vi "스마트 공장_프로젝트_3조.vi"() -> ()   [LabVIEW 2021]
uses:
  <vilib>/Utility/sysdir.llb/System Directory Type.ctl
  <vilib>/DAQmx/read.llb/DAQmx Read (Counter DBL 1Chan 1Samp).vi
  <vilib>/DAQmx/read.llb/DAQmx Read (Analog 1D Wfm NChan NSamp).vi
  <vilib>/Analysis/baseanly.llb/Mean (DBL).vi
  <vilib>/DAQmx/write.llb/DAQmx Write (Counter Frequency 1Chan 1Samp).vi
  <vilib>/DAQmx/create/channels.llb/DAQmx Create Channel (AI-Voltage-Basic).vi
  <vilib>/DAQmx/configure/timing.llb/DAQmx Timing (Sample Clock).vi
  <vilib>/DAQmx/create/channels.llb/DAQmx Create Channel (CI-Count Edges).vi
  <vilib>/DAQmx/create/channels.llb/DAQmx Create Channel (CO-Pulse Generation-Frequency).vi
  <vilib>/DAQmx/configure/timing.llb/DAQmx Timing (Implicit).vi
  <vilib>/DAQmx/miscellaneous.llb/DAQmx Fill In Error Info.vi
  <vilib>/measure/maspectr.llb/FFT Power Spectrum for N Chan.vi
  <resource>/objmgr/daqmx.rc
  <vilib>/measure/NI_MAPro.lvlib
  <vilib>/Analysis/NI_AALBase.lvlib
panel:
  in  "Axis_Factor":u16(ring) items=["X", "Y", "Z"]
  out "시간 문자열":string
  out "Temp":dbl format="%0.2f"
  out "Distance":dbl caption="DISTANCE" format="%0.2f"
  out "Z":dbl format="%0.2f"
  out "Y":dbl format="%0.2f"
  out "X":dbl format="%0.2f"
  out "t0":timestamp
  out "추가된 배열":waveform(dbl)[](array[waveform])
  out "크기":i32
  out "배열":waveform(dbl)[](array[waveform])
  out "MAX-DISTANCE":dbl
  out "웨이브폼 그래프":cluster{"f0":dbl, "df":dbl, "magnitude":dbl[]}[](graph)
  out "data":dbl caption="RPM" format="%0.2f"
  out "CONNECT":bool
  in  "stop":bool
  in  "start":bool
  in  "exit":bool
  in  "File Name":string
  in  "LIMITED-DISTANCE":dbl
  in  "디스플레이 영역(s)":dbl
  in  "Window":u16(ring)
  in  "Number of average":u16(ring)
  in  "Average mode":u16(ring)
  in  "회전당 펄스":dbl
  in  "TEMP-OFFSET":dbl
  in  "TEMP-FACTOR":dbl
  in  "DISTANCE-OFFSET":dbl
  in  "DISTANCE-FACTOR":dbl
  in  "AXIS-OFFSET":dbl
  out "웨이브폼 차트":waveform(dbl)[](graph)
  # "SMART-FACTORY"
  # "Time Domain Graph"
  # "Frequency Domain Graph"
  # "SETTING"
  # "DATA"
  # "Time Domain"
  # "Waveform graph"
  # "Time domain vertical bar"
  # "Frequency Domain"
  # "Window"
  # "Average Parameter"
  # "config data"
  # "calibration"
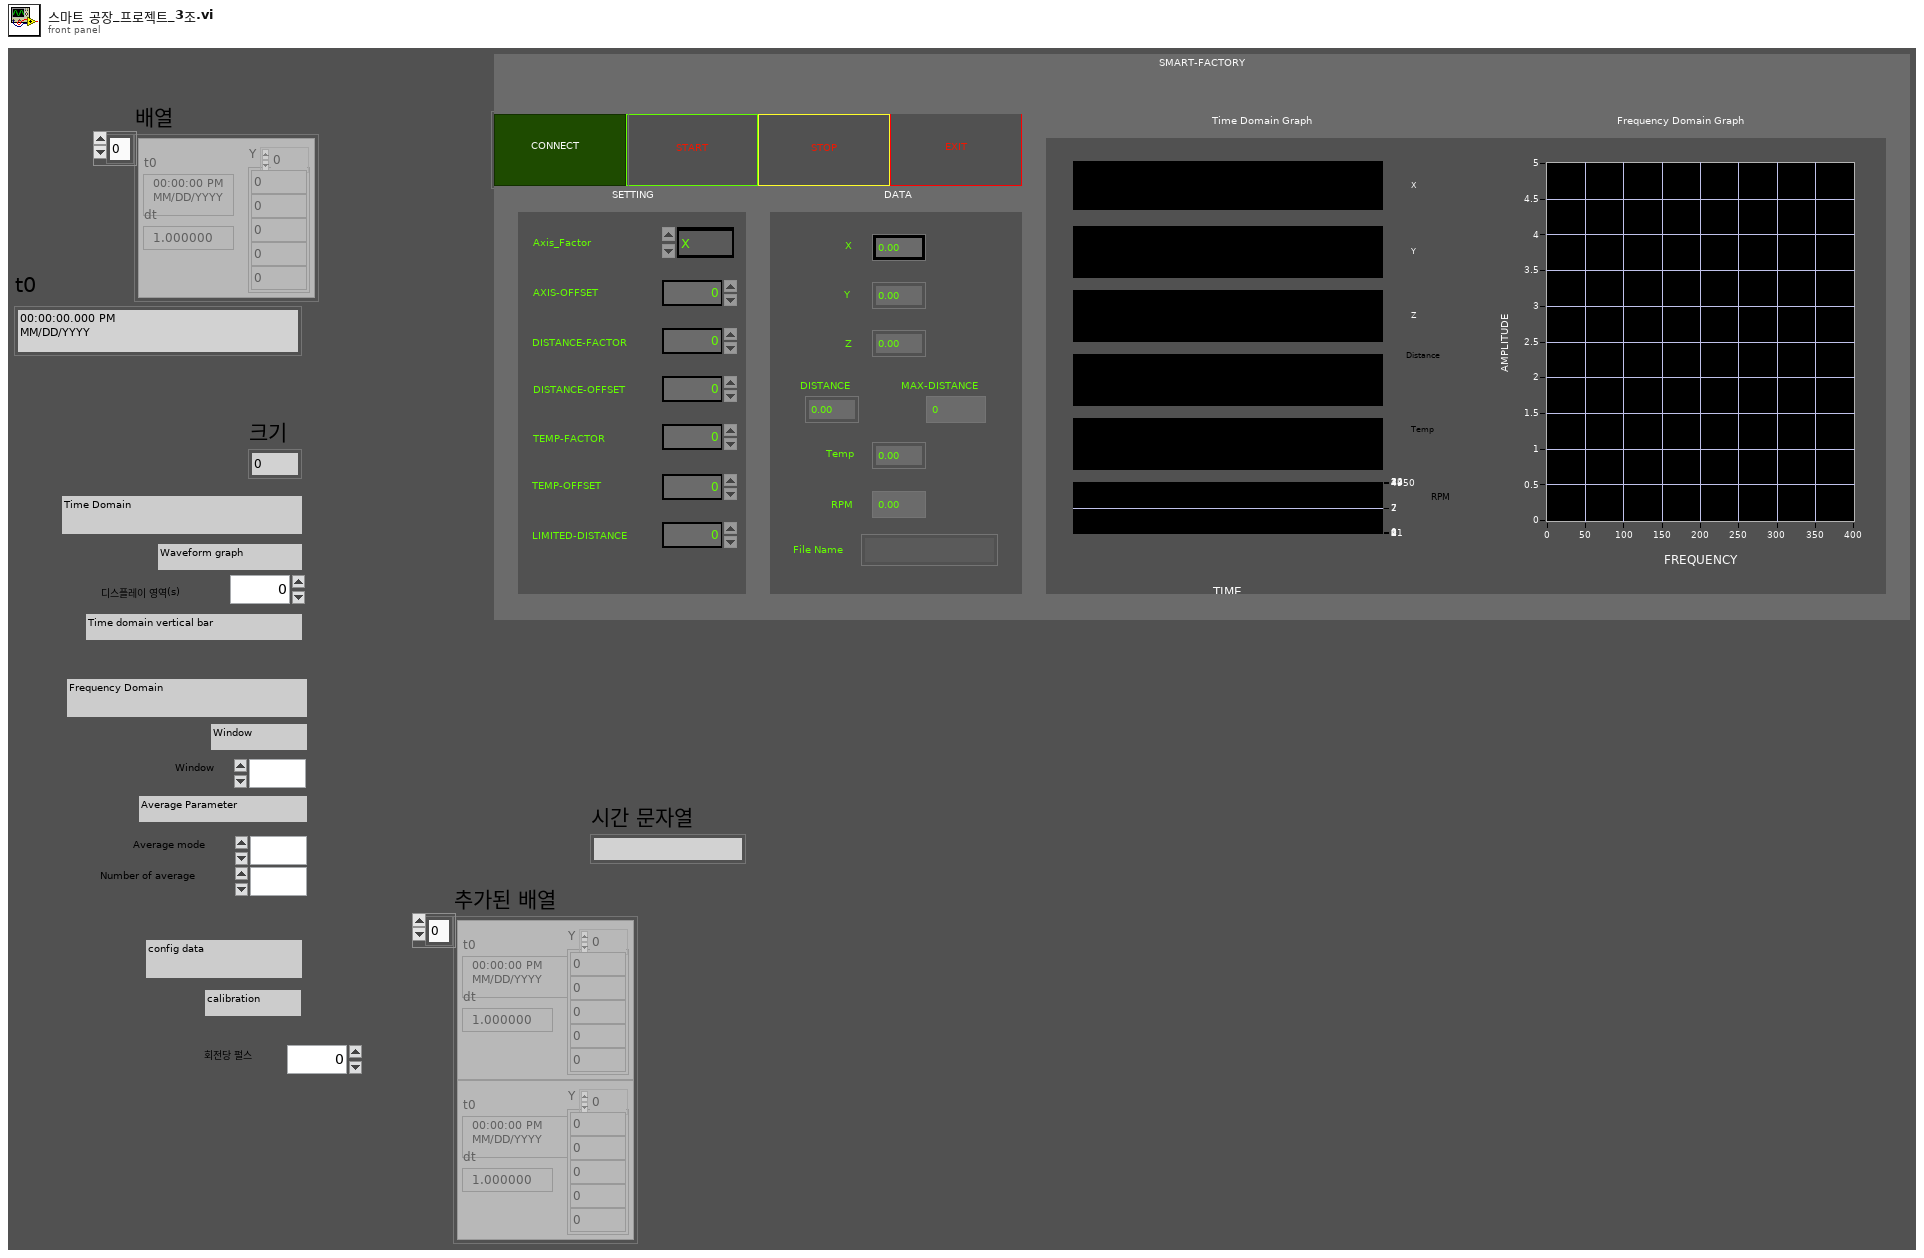
[diagram p1: front panel]
types:
  T1 = typedef "공장.ctl" = enum16{"초기화", "Ready", "Start", "Stop", "Exit"}
  T2 = cluster{"x_time(s)":i32, "y_time(s)":i32, "z_time(s)":i32, T1, "temp_time(s)":i32, "rpm_time(s)":i32, "x_data":i32, "y_data":i32, "z_data":i32, "distance_time(s)":i32, "temp_data":i32, "rpm_data":i32, "distance_data":i32, "MOTOR_PULSE":refnum<k21>, "AI_SIGNAL":refnum<k21>, "DI_SIGNAL":refnum<k21>, "CONNECT_LED":bool, "저장 파일":refnum<k34>, "system":bool, "카운트":dbl}
  T3 = enum16{"open", "open or create", "create or replace", "create", "open (read-only)"}
  T4 = enum8{"Enabled", "Disabled", "Disabled and Grayed Out"}
  T5 = typedef "System Directory Type.ctl" = i32
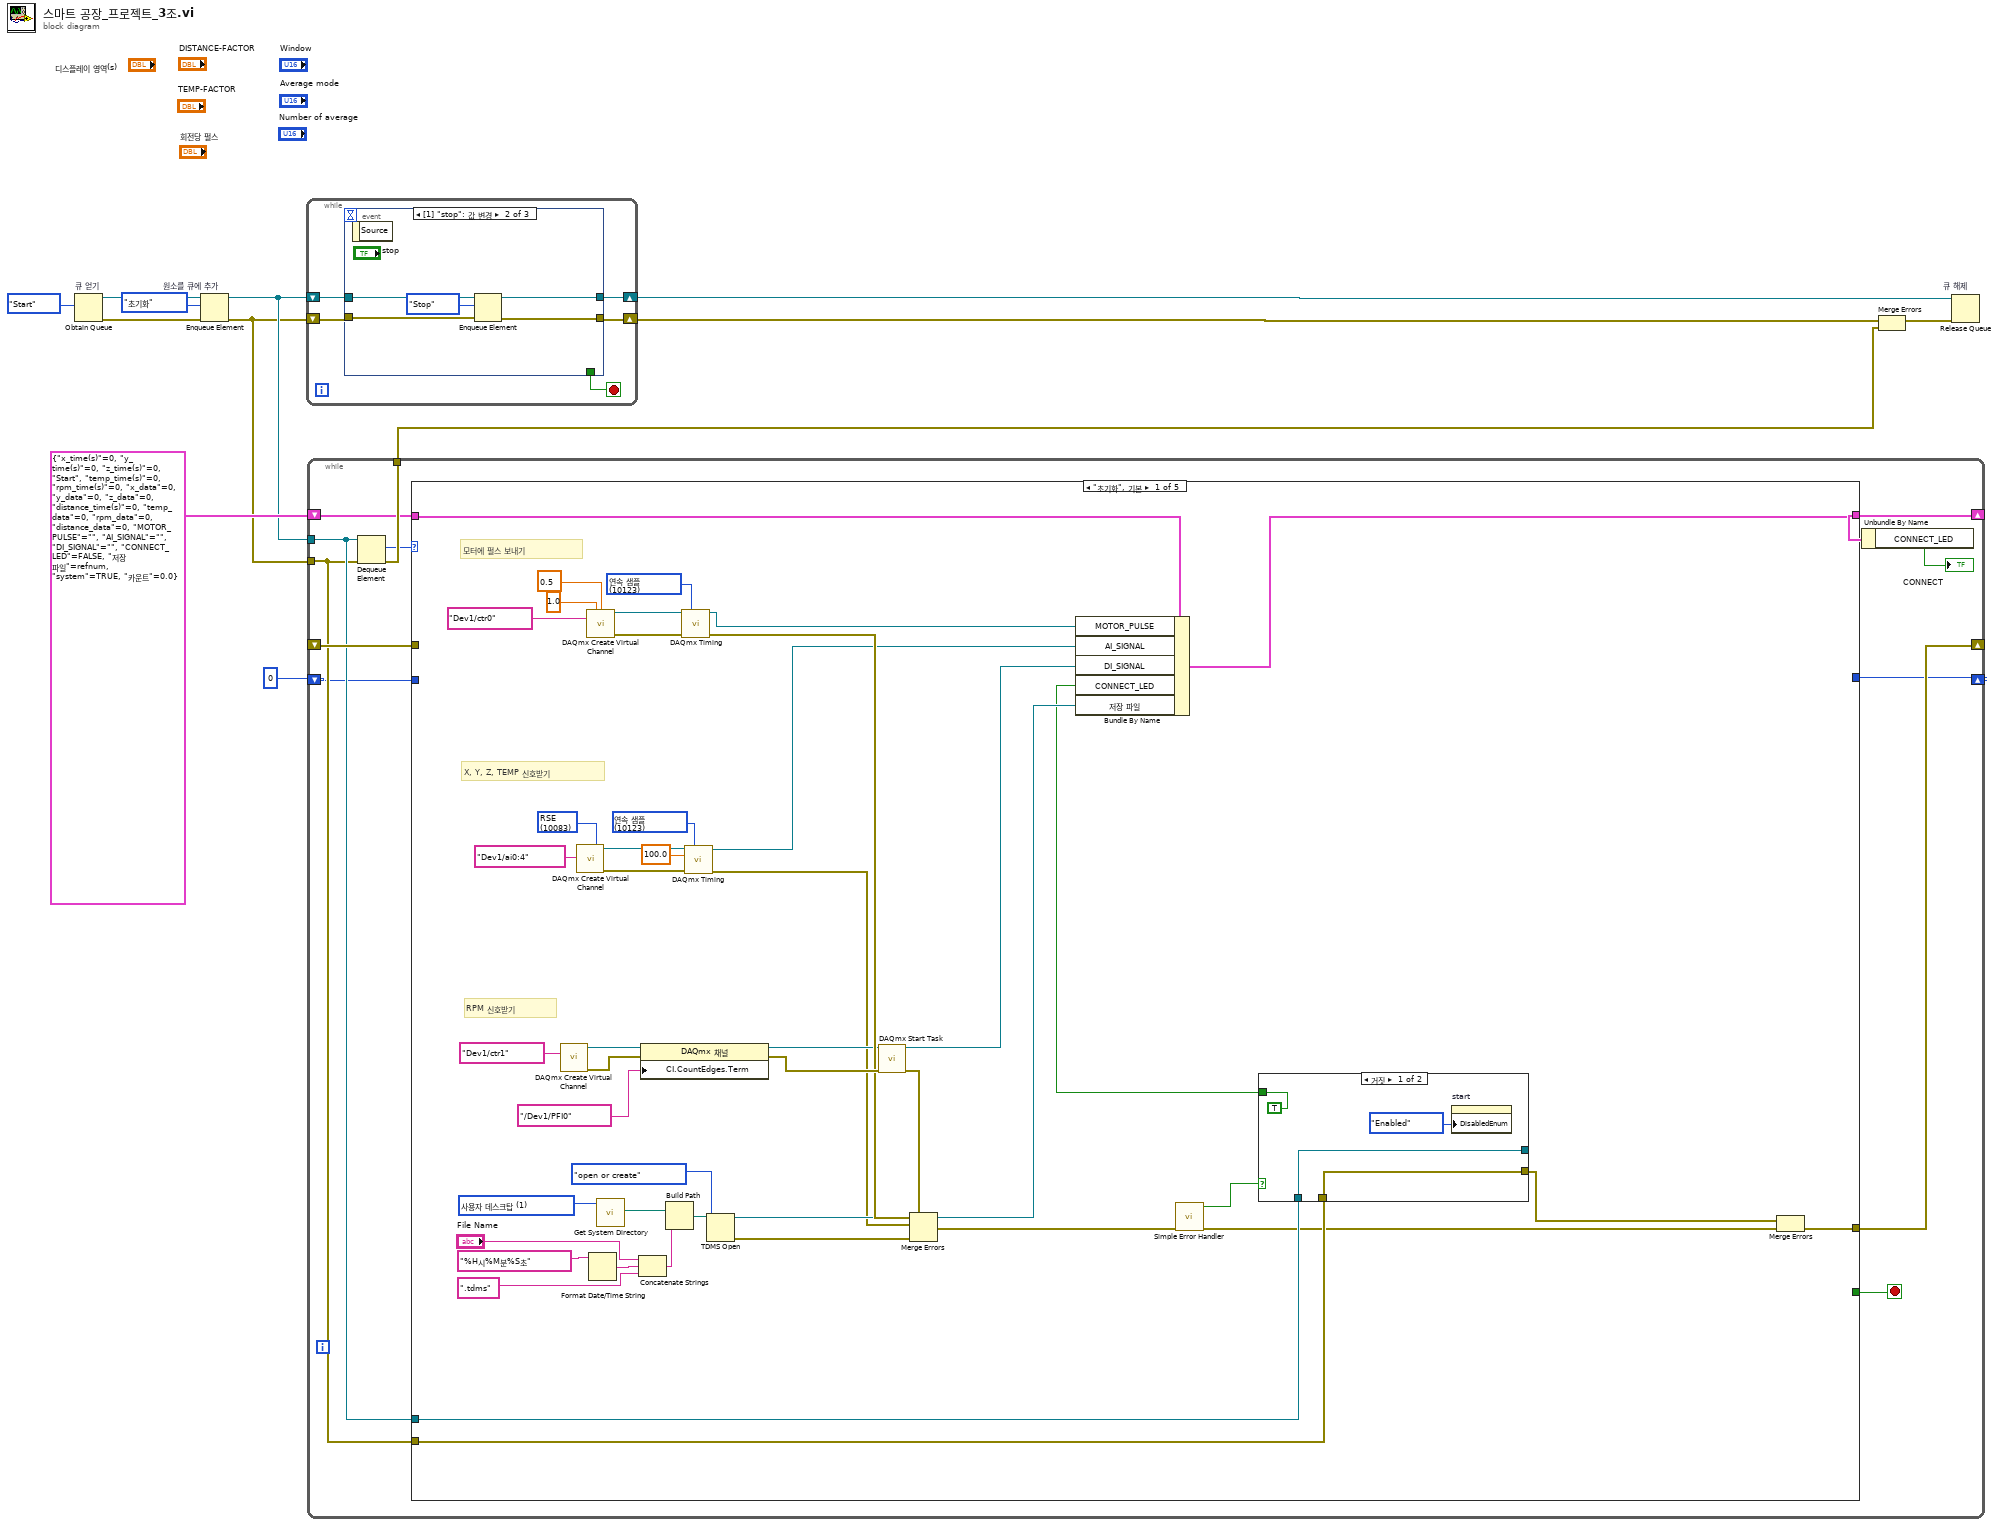
[diagram p0: block diagram]
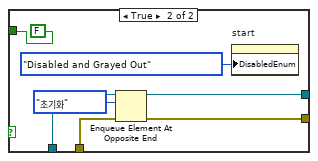
[diagram p2: hidden frame]
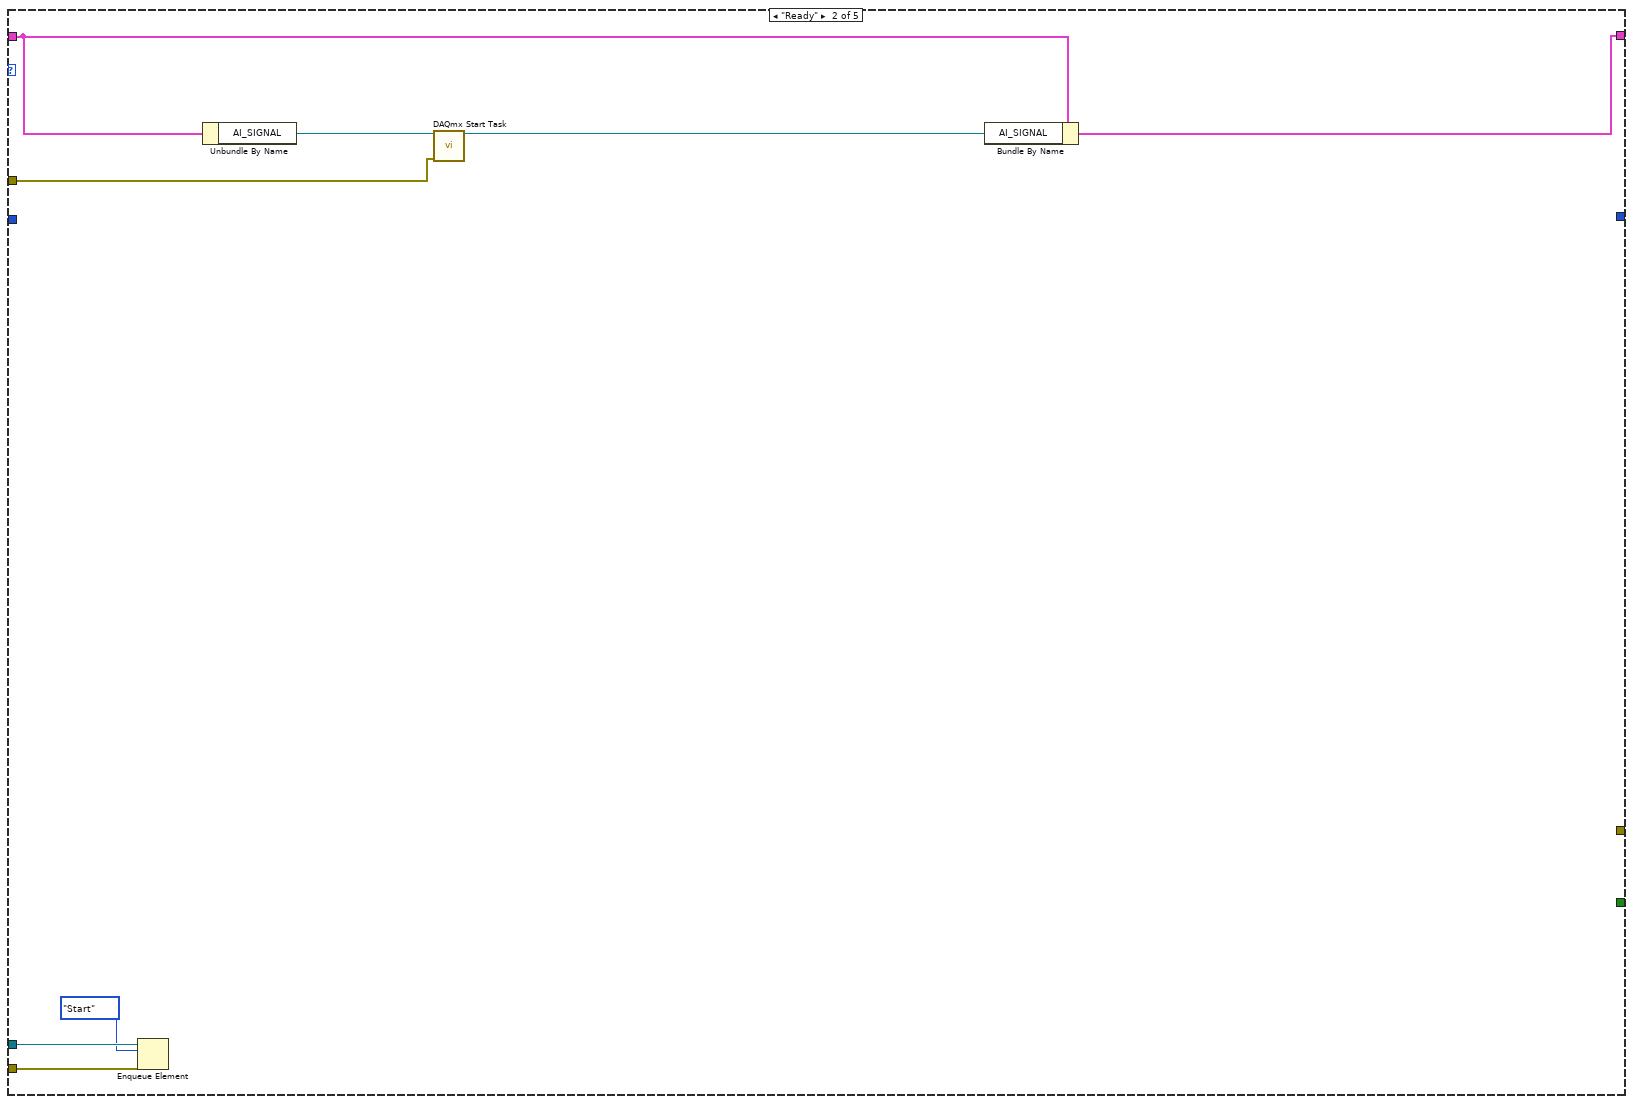
[diagram p3: hidden frame]
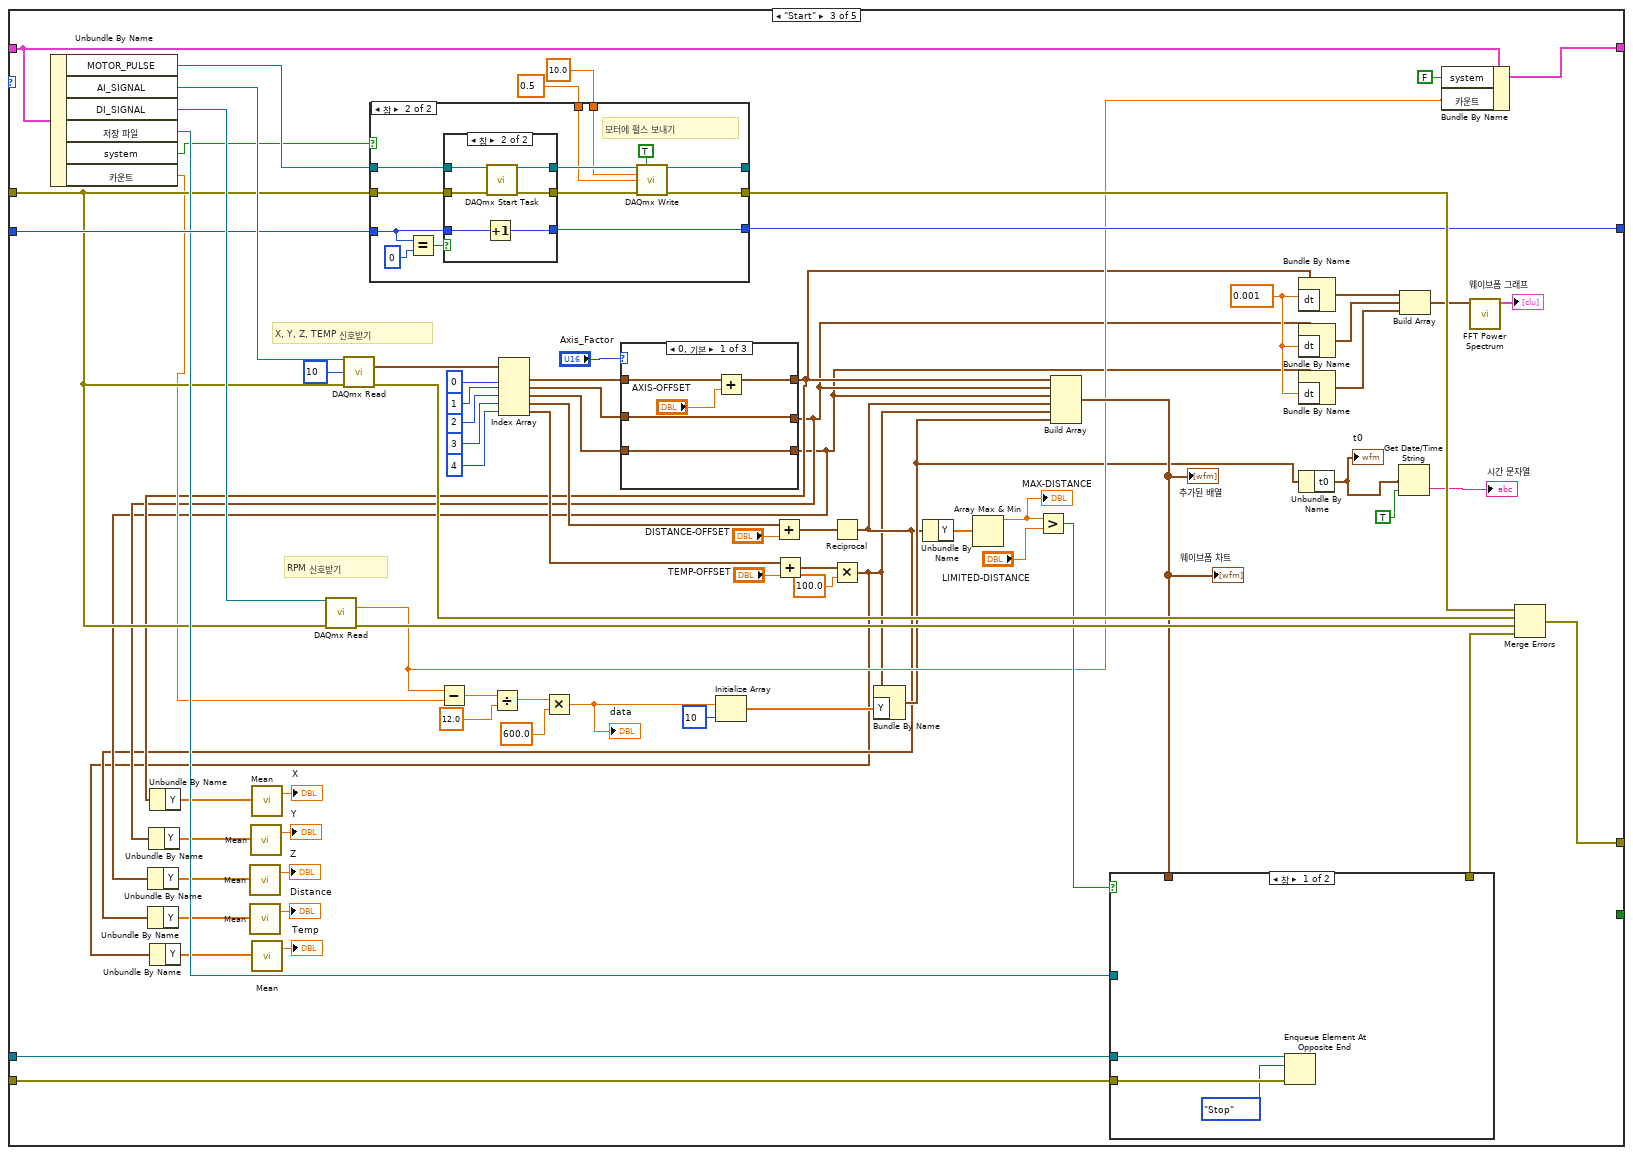
[diagram p4: hidden frame]
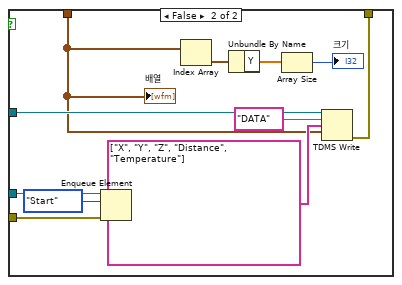
[diagram p7: hidden frame]
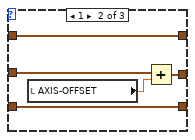
[diagram p8: hidden frame]
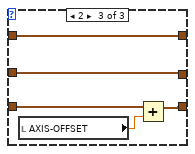
[diagram p9: hidden frame]
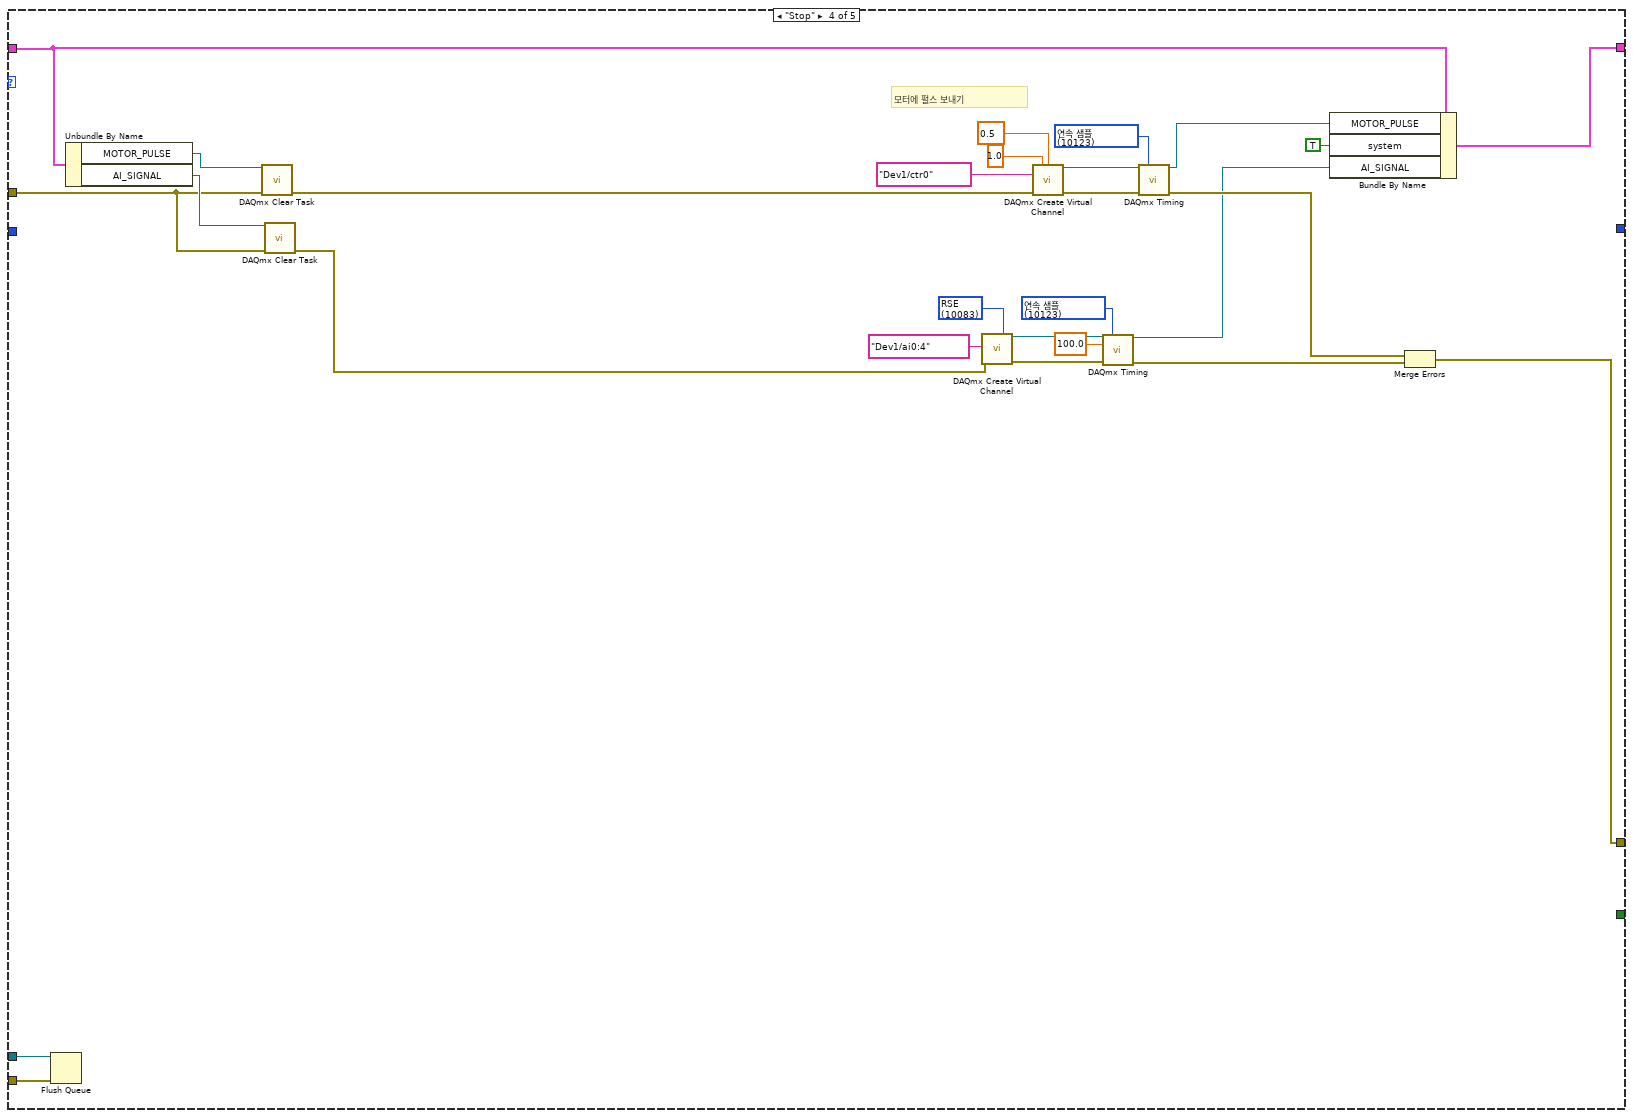
[diagram p10: hidden frame]
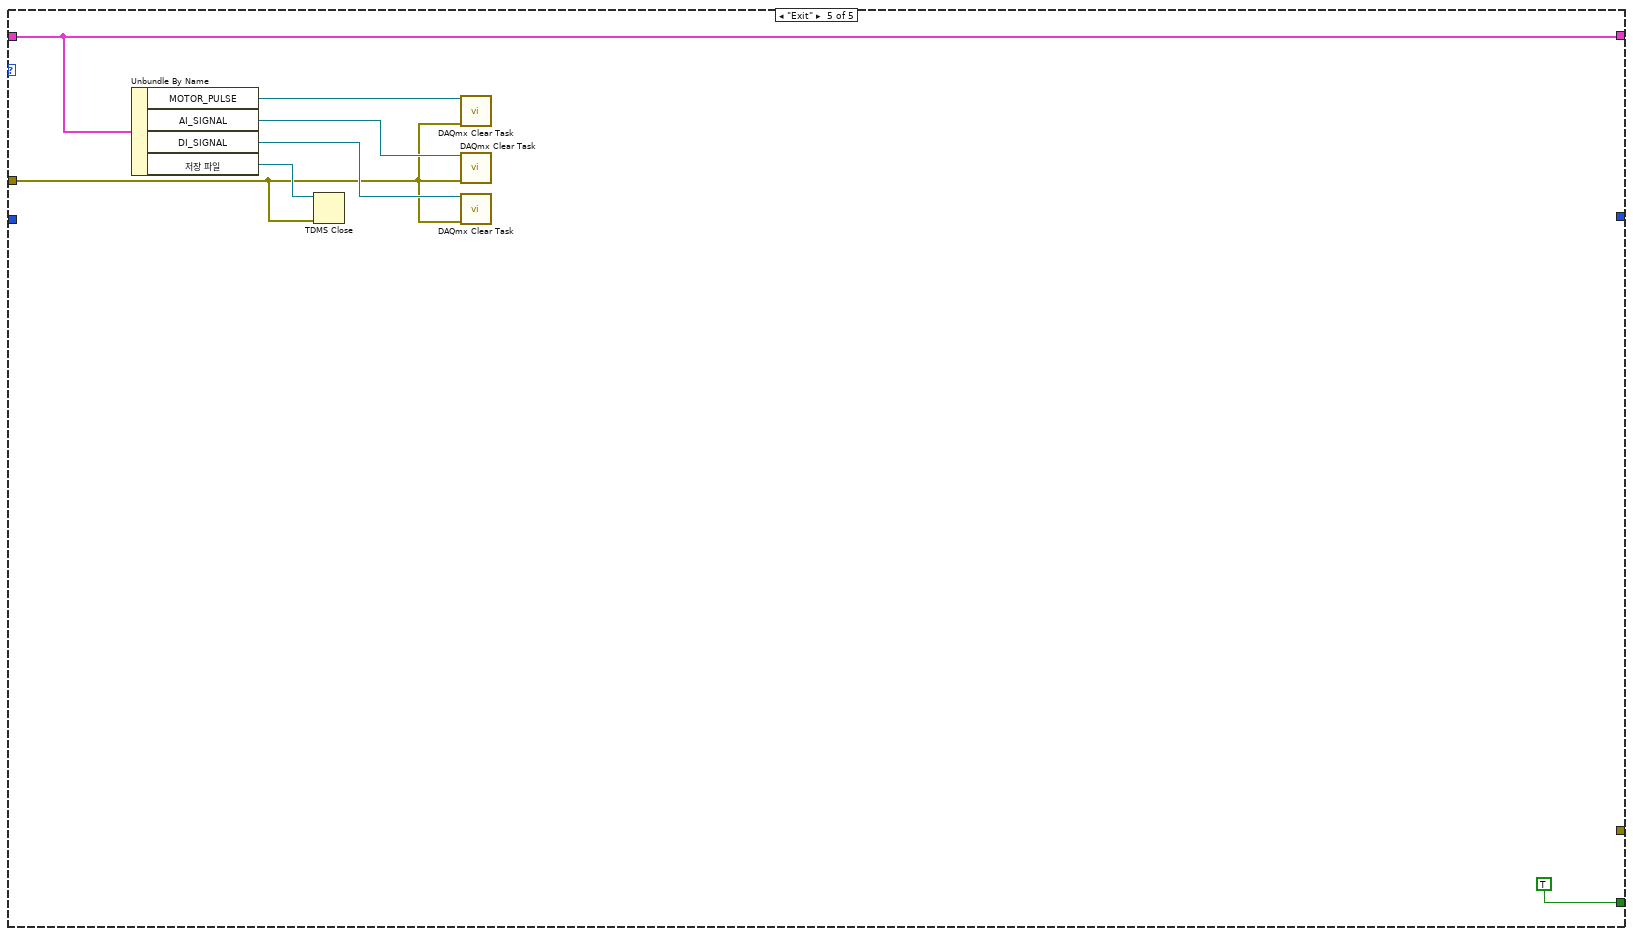
[diagram p11: hidden frame]
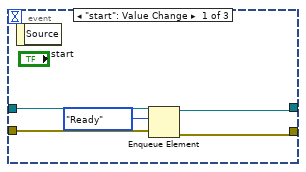
[diagram p12: hidden frame]
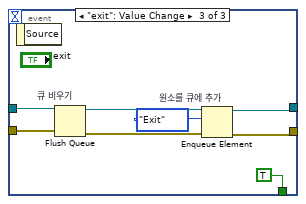
[diagram p13: hidden frame]
diagram:
  n1 = Obtain Queue "큐 얻기"(element data type=공장."Start") -> (queue out=w12:refnum<queue>, error out=w10:errorcluster)  [unwired: 4 in, 1 out]
  n2 = Enqueue Element "원소를 큐에 추가"(queue=w12, element=공장."초기화" ("원소"), error in (no error)=w10) -> (queue out=w2:refnum<queue>, error out=w1:errorcluster)  [unwired: 1 in, 1 out]
  n3 = while {
    shift-right: [w13] -> w8
    shift-left: w2 -> [w16]
    shift-right: [w15] -> w7
    shift-left: w1 -> [w14]
    stop <- w17 stop-if-true
    n4 = event shown="[1] \"stop\": 값 변경" {
      selector: _ -> [_ _ _]
      dyn-events: _ -> [_ _ _]
      timeout: _ -> [_ _ _]
      tunnel: [_ _ TRUE] -> w17
      tunnel: w16 -> [w21 w26 w31]
      tunnel: [w19 w23 w29] -> w13
      tunnel: w14 -> [w20 w25 w30]
      tunnel: [w18 w24 w28] -> w15
      event "start": Value Change {
        n5 = event-data() -> ()  [unwired: 1 in, 1 out]
        n6 = Enqueue Element(queue=w21, element=공장."Ready" ("원소"), error in (no error)=w20) -> (queue out=w19:refnum<queue>, error out=w18:errorcluster)  [unwired: 1 in, 1 out]
      }
      event "stop": Value Change {
        n7 = event-data() -> ()  [unwired: 1 in, 1 out]
        n8 = Enqueue Element(queue=w26, element=공장."Stop" ("원소"), error in (no error)=w25) -> (queue out=w23:refnum<queue>, error out=w24:errorcluster)  [unwired: 1 in, 1 out]
      }
      event "exit": Value Change {
        n9 = event-data() -> ()  [unwired: 1 in, 1 out]
        n10 = Flush Queue "큐 비우기"(queue=w31, error in (no error)=w30) -> (queue out=w34:refnum<queue>, error out=w33:errorcluster)  [unwired: 1 out]
        n11 = Enqueue Element "원소를 큐에 추가"(queue=w34, element=공장."Exit" ("원소"), error in (no error)=w33) -> (queue out=w29:refnum<queue>, error out=w28:errorcluster)  [unwired: 1 in, 1 out]
      }
    }
  }
  n12 = while {
    tunnel: w2 -> [w42]
    tunnel: w1 -> [w41]
    tunnel: [w47] -> w5
    shift-right: [w40] -> _
    shift-left: T2 {"x_time(s)"=0, "y_time(s)"=0, "z_time(s)"=0, enum."Start", "temp_time(s)"=0, "rpm_time(s)"=0, "x_data"=0, "y_data"=0, "z_data"=0, "distance_time(s)"=0, "temp_data"=0, "rpm_data"=0, "distance_data"=0, "MOTOR_PULSE"="", "AI_SIGNAL"="", "DI_SIGNAL"="", "CONNECT_LED"=FALSE, "저장 파일"=refnum, "system"=TRUE, "카운트"=0.0} -> [w45]
    shift-right: [w44] -> _
    shift-left: _ -> [w43]
    shift-right: [w37] -> _
    shift-left: 0 -> [w38]
    stop <- w46 stop-if-true
    n13 = Dequeue Element ("원소를 큐에서 제거")(queue=w42, error in (no error)=w41) -> (element=w36:T1, error out=w47:errorcluster)  [unwired: 1 in, 2 out]
    n14 = case shown="\"초기화\", 기본" w36 {
      tunnel: [_ _ _ _ TRUE] -> w46
      tunnel: [w62 w107 w145 w259 w275] -> w40
      tunnel: w45 -> [w63 w109 w146 w260 w275]
      tunnel: [w54 _ w149 w247 _] -> w44
      tunnel: w43 -> [_ w110 w150 w255 w270]
      tunnel: w42 -> [w55 w106 w171 w269 _]
      tunnel: w41 -> [w56 w105 w170 w268 _]
      tunnel: w38 -> [_ _ w168 _ _]
      tunnel: [_ _ w167 _ _] -> w37
      frame "초기화", Default {
        w74 = T5 1 items=["사용자 홈"=0, "사용자 데스크탑"=1, "사용자 문서"=2, "사용자 어플리케이션 데이터"=3, "사용자 환경"=4, "사용자 임시"=5, "퍼블릭 문서"=6, "퍼블릭 어플리케이션 데이터"=7, "퍼블릭 환경"=8, "퍼블릭 캐시"=13, "시스템 코어 라이브러리"=9, "시스템 설치된 라이브러리"=10, "어플리케이션 파일"=11, "부팅 볼륨 루트"=12] ("system directory type")
        w85 = 10123 items=["유한 샘플"=10178, "연속 샘플"=10123, "하드웨어 타이밍에 의한 단일 포인트"=12522] ("sample mode")
        w88 = 10083 items=["기본"=-1, "RSE"=10083, "NRSE"=10078, "차동"=10106, "유사 차동"=12529] ("input terminal configuration")
        w90 = 10123 items=["유한 샘플"=10178, "연속 샘플"=10123, "하드웨어 타이밍에 의한 단일 포인트"=12522] ("sample mode")
        # "RPM 신호받기"
        # "X, Y, Z, TEMP 신호받기"
        # "모터에 펄스 보내기"
        n15 = call-poly <vilib>:"DAQmx Create Virtual Channel.vi"("counter"=tag "Dev1/ctr1") -> ("task out"=w81:refnum<k21>, "error out"=w80:errorcluster)  [unwired: 13 in]
        n16 = call-poly <vilib>:"DAQmx Create Virtual Channel.vi"("input terminal configuration"=w88, "physical channels"=tag "Dev1/ai0:4") -> ("task out"=w87:refnum<k21>, "error out"=w86:errorcluster)  [unwired: 12 in]
        n17 = call-poly <vilib>:"DAQmx Create Virtual Channel.vi"("frequency"=1.0, "duty cycle"=0.5, "counter"=tag "Dev1/ctr0") -> ("task out"=w67:refnum<k21>, "error out"=w89:errorcluster)  [unwired: 11 in]
        n18 = Format Date/Time String(time format string (%c)="%H시%M분%S초" ("시간 포맷 문자열 (%c)")) -> (date/time string=w59:string)  [unwired: 2 in]
        n19 = call <vilib>:"Get System Directory.vi"("system directory type"=w74) -> ("system directory"=w73:path)  [unwired: 10 in]
        n20 = Concatenate Strings("File Name", w59, ".tdms" ("문자열")) -> (w58:string)
        n21 = property class="DAQmx 채널"(reference=w81, error in=w80, "CI.CountEdges.Term"=tag "/Dev1/PFI0" ("카운터 입력:주파수:입력:터미널")) -> (reference out=w66:refnum<k21>, error out=w79:errorcluster)
        n22 = Build Path(base path=w73, name or relative path=w58) -> (appended path=w72:path)
        n23 = call-poly <vilib>:"DAQmx Timing.vi"("task/channels in"=w67, "sample mode"=w90, "error in"=w89) -> ("task out"=w76:refnum<k21>, "error out"=w75:errorcluster)  [unwired: 11 in]
        n24 = call-poly <vilib>:"DAQmx Timing.vi"("task/channels in"=w87, "sample mode"=w85, "rate"=100.0, "error in"=w86) -> ("task out"=w50:refnum<k21>, "error out"=w49:errorcluster)  [unwired: 10 in]
        n25 = TDMS Open(10:T3."open or create" ("동작(0:open)"), 11:w72) -> (0:w70:errorcluster, 3:w71:refnum<k34>)  [unwired: 5 in]
        n26 = call <vilib>:"DAQmx Start Task.vi"("task/channels in"=w66, "error in"=w79) -> ("task out"=w65:refnum<k21>, "error out"=w78:errorcluster)  [unwired: 12 in]
        n27 = Merge Errors(w75, w49, w78, w70) -> (w77:errorcluster)
        n28 = call <vilib>:"Simple Error Handler.vi"("error in (no error)"=w77) -> ("error?"=w53:bool, "error out"=w52:errorcluster)  [unwired: 4 in, 3 out]
        n29 = case shown="거짓" w53 {
          tunnel: w56 -> [w94 w102]
          tunnel: w55 -> [w93 w101]
          tunnel: [w94 w100] -> w48
          tunnel: [TRUE ("CONNECT_LED") FALSE] -> w51
          tunnel: [w93 w97] -> _
          frame False {
            n30 = property on="start" class="Bool"("DisabledEnum"=T4."Enabled" ("비활성화")) -> ()  [unwired: 2 in, 2 out]
          }
          frame True {
            n31 = Enqueue Element At Opposite End(queue=w101, element=공장."초기화" ("원소"), error in (no error)=w102) -> (queue out=w97:refnum<queue>, error out=w100:errorcluster)  [unwired: 1 in, 1 out]
            n32 = property on="start" class="Bool"("DisabledEnum"=T4."Disabled and Grayed Out" ("비활성화")) -> ()  [unwired: 2 in, 2 out]
          }
        }
        n33 = Bundle By Name(cluster=w63, "MOTOR_PULSE"=w76, "AI_SIGNAL"=w50, "DI_SIGNAL"=w65, "CONNECT_LED"=w51, "저장 파일"=w71) -> (w62:T2)
        n34 = Merge Errors(w48, w52) -> (w54:errorcluster)
      }
      frame "Ready" {
        n35 = Enqueue Element(queue=w106, element=공장."Start" ("원소"), error in (no error)=w105) -> ()  [unwired: 1 in, 3 out]
        n36 = Unbundle By Name(w109) -> ("AI_SIGNAL"=w111:refnum<k21>)
        n37 = call <vilib>:"DAQmx Start Task.vi"("task/channels in"=w111, "error in"=w110) -> ("task out"=w108:refnum<k21>)  [unwired: 12 in, 1 out]
        n38 = Bundle By Name(cluster=w109, "AI_SIGNAL"=w108) -> (w107:T2)
      }
      frame "Start" {
        w148 = 0.001 ("dt")
        # "RPM 신호받기"
        # "X, Y, Z, TEMP 신호받기"
        n39 = Unbundle By Name(w146) -> ("MOTOR_PULSE"=w169:refnum<k21>, "AI_SIGNAL"=w188:refnum<k21>, "DI_SIGNAL"=w187:refnum<k21>, "저장 파일"=w155:refnum<k34>, "system"=w147:bool, "카운트"=w141:dbl)
        n40 = call-poly <vilib>:"DAQmx Read.vi"("task/channels in"=w187, "error in"=w150) -> ("data"=w142:dbl, "error out"=w184:errorcluster)  [unwired: 11 in, 1 out]
        n41 = call-poly <vilib>:"DAQmx Read.vi"("task/channels in"=w188, "number of samples per channel"=10, "error in"=w150) -> ("data"=w175:waveform(dbl)[], "error out"=w185:errorcluster)  [unwired: 10 in, 1 out]
        n42 = case shown="참" w147 {
          tunnel: w169 -> [w191 w197]
          tunnel: w150 -> [w190 w195]
          tunnel: [w191 w203] -> _
          tunnel: [w190 w202] -> w186
          tunnel: w168 -> [w189 w200]
          tunnel: [w189 w201] -> w167
          tunnel: 10.0 ("frequency") -> [_ w193]
          tunnel: 0.5 ("duty cycle") -> [_ w192]
          frame False {
          }
          frame True {
            # "모터에 펄스 보내기"
            n43 = Equal?(x=w200, y=0) -> (x = y?=w198:bool)
            n44 = case shown="참" w198 {
              tunnel: w200 -> [w207 w213]
              tunnel: [w207 w212] -> w201
              tunnel: w197 -> [w205 w211]
              tunnel: [w205 w210] -> w196
              tunnel: [w206 w209] -> w194
              tunnel: w195 -> [w206 w208]
              frame False {
              }
              frame True {
                n45 = Increment(x=w213) -> (x+1=w212:i32)
                n46 = call <vilib>:"DAQmx Start Task.vi"("task/channels in"=w211, "error in"=w208) -> ("task out"=w210:refnum<k21>, "error out"=w209:errorcluster)  [unwired: 12 in]
              }
            }
            n47 = call-poly <vilib>:"DAQmx Write.vi"("task/channels in"=w196, "auto start"=TRUE, "frequency"=w193, "duty cycle"=w192, "error in"=w194) -> ("task out"=w203:refnum<k21>, "error out"=w202:errorcluster)  [unwired: 8 in, 1 out]
          }
        }
        n48 = Subtract(x=w142, y=w141) -> (x-y=w140:dbl)
        n49 = Divide(x=w140, y=12.0) -> (x/y=w138:dbl)
        n50 = Index Array(array=w175, index #1=0 ("인덱스 (행)"), index #2=1 ("인덱스"), index #3=2 ("인덱스"), index #4=3 ("인덱스"), index #5=4) -> (element #1=w177:waveform(dbl), element #2=w163:waveform(dbl), element #3=w162:waveform(dbl), element #4=w161:waveform(dbl), element #5=w160:waveform(dbl))
        n51 = Multiply(x=w138, y=600.0) -> (x*y=w136:dbl)
        "data" <- w136
        n52 = case shown="0, 기본" "Axis_Factor" {
          tunnel: w177 -> [w232 w236 w242]
          tunnel: [w231 w236 w242] -> w131
          tunnel: [w229 w233 w241] -> w129
          tunnel: w163 -> [w229 w234 w241]
          tunnel: w162 -> [w228 w237 w239]
          tunnel: [w228 w237 w238] -> w128
          frame 0, Default {
            n53 = Add(x=w232, y="AXIS-OFFSET") -> (x+y=w231:waveform(dbl))
          }
          frame 1 {
            n54 = local read "AXIS-OFFSET"() -> (w235:dbl)
            n55 = Add(x=w234, y=w235) -> (x+y=w233:waveform(dbl))
          }
          frame 2 {
            n56 = local read "AXIS-OFFSET"() -> (w240:dbl)
            n57 = Add(x=w239, y=w240) -> (x+y=w238:waveform(dbl))
          }
        }
        n58 = Unbundle By Name(w128) -> ("Y"=w124:dbl[])
        n59 = Unbundle By Name(w129) -> ("Y"=w125:dbl[])
        n60 = Unbundle By Name(w131) -> ("Y"=w130:dbl[])
        n61 = call-poly <vilib>:"Mean.vi"("X"=w124) -> ("mean"=→"Z":dbl)  [unwired: 1 out]
        n62 = call-poly <vilib>:"Mean.vi"("X"=w125) -> ("mean"=→"Y":dbl)  [unwired: 1 out]
        n63 = call-poly <vilib>:"Mean.vi"("X"=w130) -> ("mean"=→"X":dbl)  [unwired: 1 out]
        n64 = Initialize Array(w136, 10 ("차원 크기")) -> (w134:dbl[])
        n65 = Add(x=w161, y="DISTANCE-OFFSET") -> (x+y=w158:waveform(dbl))
        n66 = Add(x=w160, y="TEMP-OFFSET") -> (x+y=w157:waveform(dbl))
        n67 = Reciprocal(x=w158) -> (1/x=w127:waveform(dbl))
        n68 = Unbundle By Name(w127) -> ("Y"=w123:dbl[])
        n69 = call-poly <vilib>:"Mean.vi"("X"=w123) -> ("mean"=→"Distance":dbl)  [unwired: 1 out]
        n70 = Multiply(x=w157, y=100.0) -> (x*y=w126:waveform(dbl))
        n71 = Unbundle By Name(w126) -> ("Y"=w122:dbl[])
        n72 = call-poly <vilib>:"Mean.vi"("X"=w122) -> ("mean"=→"Temp":dbl)  [unwired: 1 out]
        n73 = Bundle By Name(cluster=w126, "Y"=w134) -> (w133:waveform(dbl))
        n74 = Unbundle By Name(w127) -> ("Y"=w113:dbl[])
        n75 = Array Max & Min(array=w113) -> (max value=w112:dbl)  [unwired: 3 out]
        "MAX-DISTANCE" <- w112
        n76 = Greater?(x=w112, y="LIMITED-DISTANCE") -> (0:w172:bool)
        n77 = Build Array ("배열 만들기")(w131, w129, w128, w127, w126, w133) -> (w153:waveform(dbl)[])
        "웨이브폼 차트" <- w153
        "추가된 배열" <- w153
        n78 = case shown="참" w172 {
          tunnel: w171 -> [w216 w227]
          tunnel: w170 -> [w215 w226]
          tunnel: w155 -> [_ w221]
          tunnel: [_ w222] -> w154
          tunnel: w153 -> [_ w220]
          frame True {
            n79 = Enqueue Element At Opposite End(queue=w216, element=공장."Stop" ("원소"), error in (no error)=w215) -> ()  [unwired: 1 in, 3 out]
          }
          frame False {
            n80 = Enqueue Element(queue=w227, element=공장."Start" ("원소"), error in (no error)=w226) -> ()  [unwired: 1 in, 3 out]
            n81 = Index Array(array=w220) -> (element=w219:waveform(dbl))  [unwired: 1 in]
            n82 = Unbundle By Name(w219) -> ("Y"=w218:dbl[])
            n83 = Array Size(array=w218) -> (size(s)=→"크기":i32)
            n84 = TDMS Write(0:w221, 5:"DATA" ("그룹 이름 입력(제목없음)"), 7:string[] ["X", "Y", "Z", "Distance", "Temperature"] ("채널 이름 입력(제목없음)"), 9:w220) -> (15:w222:errorcluster)  [unwired: 2 in, 3 out]
            "배열" <- w220
          }
        }
        n85 = Bundle By Name ("웨이브폼 만들기")(cluster=w131, "dt"=w148) -> (w181:waveform(dbl))
        n86 = Bundle By Name ("웨이브폼 만들기")(cluster=w129, "dt"=w148) -> (w180:waveform(dbl))
        n87 = Bundle By Name ("웨이브폼 만들기")(cluster=w128, "dt"=w148) -> (w179:waveform(dbl))
        n88 = Unbundle By Name(w133) -> ("t0"=w132:timestamp)
        "t0" <- w132
        n89 = Get Date/Time String(seconds (now)=w132, want seconds? (F)=TRUE ("초 보이기? (거짓)")) -> (time string=→"시간 문자열":string)  [unwired: 1 in, 1 out]
        n90 = Build Array(w181, w180, w179) -> (w178:waveform(dbl)[])
        n91 = Bundle By Name(cluster=w146, "system"=FALSE, "카운트"=w142) -> (w145:T2)
        n92 = call-poly <vilib>:"FFT Power Spectrum.vi"("time signals"=w178) -> ("power spectra"=→"웨이브폼 그래프":cluster{"f0":dbl, "df":dbl, "magnitude":dbl[]}[])  [unwired: 7 in, 3 out]
        n93 = Merge Errors(w186, w185, w184, w154) -> (w149:errorcluster)
      }
      frame "Stop" {
        w250 = 10123 items=["유한 샘플"=10178, "연속 샘플"=10123, "하드웨어 타이밍에 의한 단일 포인트"=12522] ("sample mode")
        w253 = 10083 items=["기본"=-1, "RSE"=10083, "NRSE"=10078, "차동"=10106, "유사 차동"=12529] ("input terminal configuration")
        w265 = 10123 items=["유한 샘플"=10178, "연속 샘플"=10123, "하드웨어 타이밍에 의한 단일 포인트"=12522] ("sample mode")
        # "모터에 펄스 보내기"
        n94 = Flush Queue(queue=w269, error in (no error)=w268) -> ()  [unwired: 3 out]
        n95 = Unbundle By Name(w260) -> ("MOTOR_PULSE"=w267:refnum<k21>, "AI_SIGNAL"=w256:refnum<k21>)
        n96 = call <vilib>:"DAQmx Clear Task.vi"("task in"=w267, "error in"=w255) -> ("error out"=w246:errorcluster)  [unwired: 13 in]
        n97 = call <vilib>:"DAQmx Clear Task.vi"("task in"=w256, "error in"=w255) -> ("error out"=w245:errorcluster)  [unwired: 13 in]
        n98 = call-poly <vilib>:"DAQmx Create Virtual Channel.vi"("input terminal configuration"=w253, "physical channels"=tag "Dev1/ai0:4", "error in"=w245) -> ("task out"=w252:refnum<k21>, "error out"=w251:errorcluster)  [unwired: 11 in]
        n99 = call-poly <vilib>:"DAQmx Create Virtual Channel.vi"("frequency"=1.0, "duty cycle"=0.5, "counter"=tag "Dev1/ctr0", "error in"=w246) -> ("task out"=w261:refnum<k21>, "error out"=w264:errorcluster)  [unwired: 10 in]
        n100 = call-poly <vilib>:"DAQmx Timing.vi"("task/channels in"=w252, "sample mode"=w250, "rate"=100.0, "error in"=w251) -> ("task out"=w244:refnum<k21>, "error out"=w243:errorcluster)  [unwired: 10 in]
        n101 = call-poly <vilib>:"DAQmx Timing.vi"("task/channels in"=w261, "sample mode"=w265, "error in"=w264) -> ("task out"=w258:refnum<k21>, "error out"=w248:errorcluster)  [unwired: 11 in]
        n102 = Bundle By Name(cluster=w260, "MOTOR_PULSE"=w258, "system"=TRUE, "AI_SIGNAL"=w244) -> (w259:T2)
        n103 = Merge Errors(w248, w243) -> (w247:errorcluster)
      }
      frame "Exit" {
        n104 = Unbundle By Name(w275) -> ("MOTOR_PULSE"=w274:refnum<k21>, "AI_SIGNAL"=w273:refnum<k21>, "DI_SIGNAL"=w272:refnum<k21>, "저장 파일"=w271:refnum<k34>)
        n105 = TDMS Close(8:w270, 11:w271) -> ()  [unwired: 2 out]
        n106 = call <vilib>:"DAQmx Clear Task.vi"("task in"=w274, "error in"=w270) -> ()  [unwired: 13 in, 1 out]
        n107 = call <vilib>:"DAQmx Clear Task.vi"("task in"=w273, "error in"=w270) -> ()  [unwired: 13 in, 1 out]
        n108 = call <vilib>:"DAQmx Clear Task.vi"("task in"=w272, "error in"=w270) -> ()  [unwired: 13 in, 1 out]
      }
    }
    n109 = Unbundle By Name(w40) -> ("CONNECT_LED"=→"CONNECT":bool)
  }
  n110 = Merge Errors(w7, w5) -> (w6:errorcluster)
  n111 = Release Queue "큐 해제"(queue=w8, error in (no error)=w6) -> ()  [unwired: 1 in, 3 out]
